vi "Test Decoding Data.vi"() -> ()   [LabVIEW 2019]
uses:
  <vilib>/Analysis/3filter.llb/Filter Passband Type.ctl
  <vilib>/Utility/file.llb/Read Delimited Spreadsheet (DBL).vi
  <vilib>/Analysis/3filter.llb/Elliptic Filter (DBL).vi
  <vilib>/Analysis/NI_AALBase.lvlib
panel:
  out "first row":dbl[](array[numeric])
  out "Rebuild values":dbl[][](array[numeric])
  out "all rows":dbl[][](array[numeric])
  out "Filtered Graph":dbl[](graph)
  in  "ch":i32=1
  out "Original Graph":dbl[](graph)
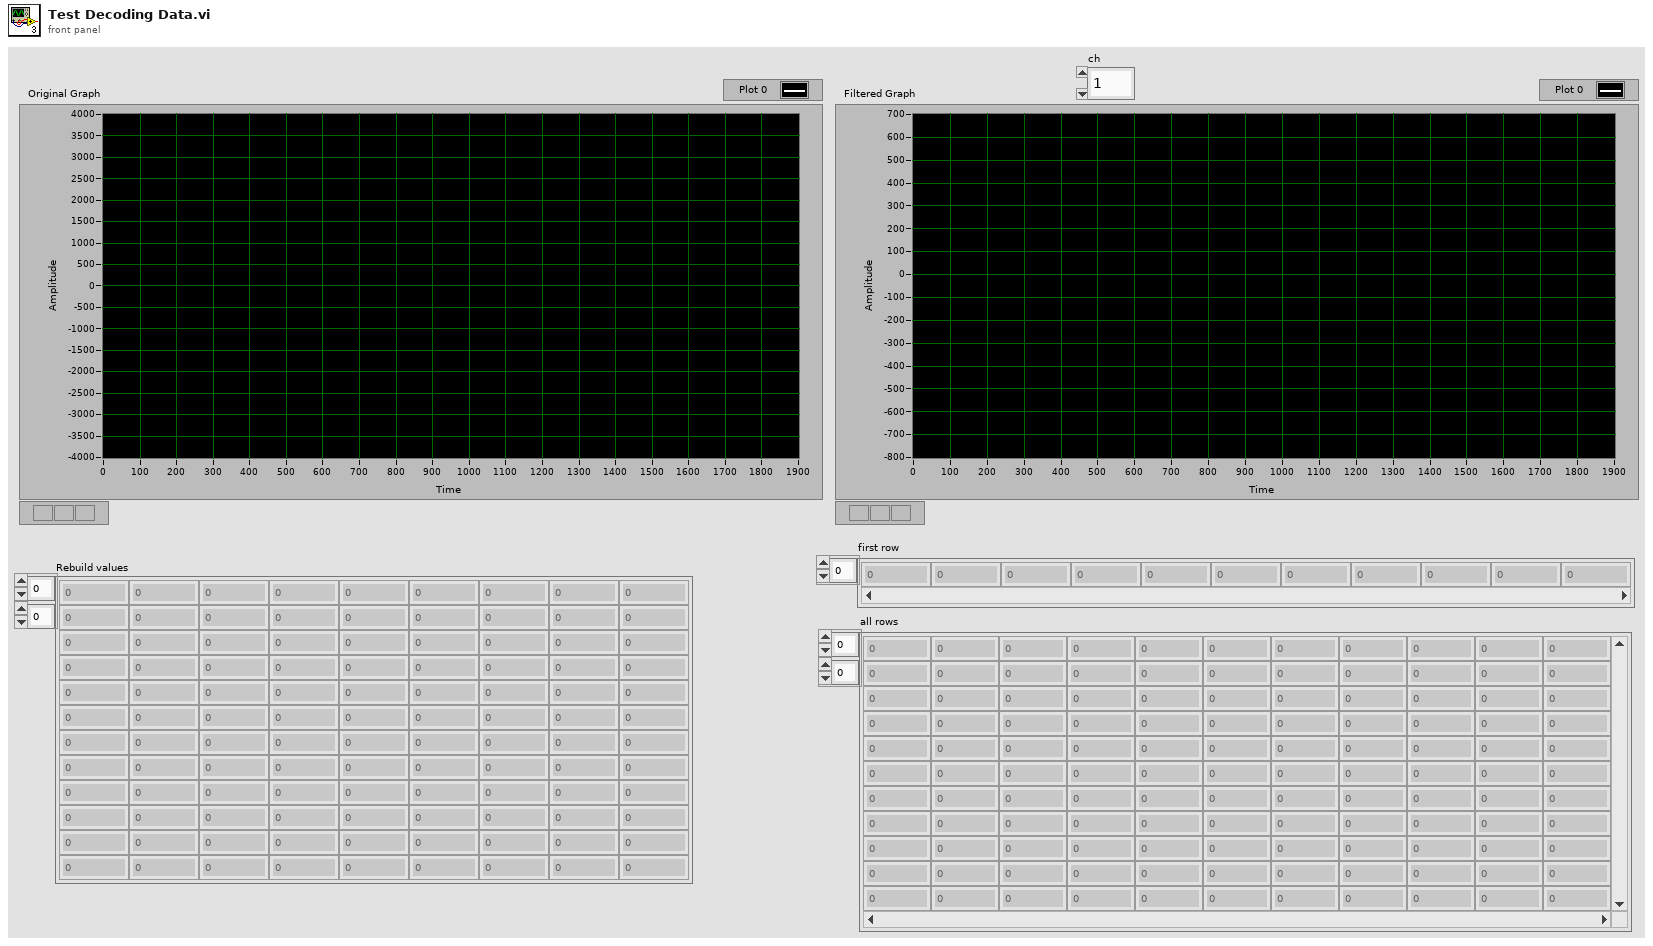
[diagram p1: front panel]
types:
  T1 = typedef "NI_AALBase.lvlib/Filter Passband Type.ctl" = enum32{"Lowpass", "Highpass", "Bandpass", "Bandstop"}
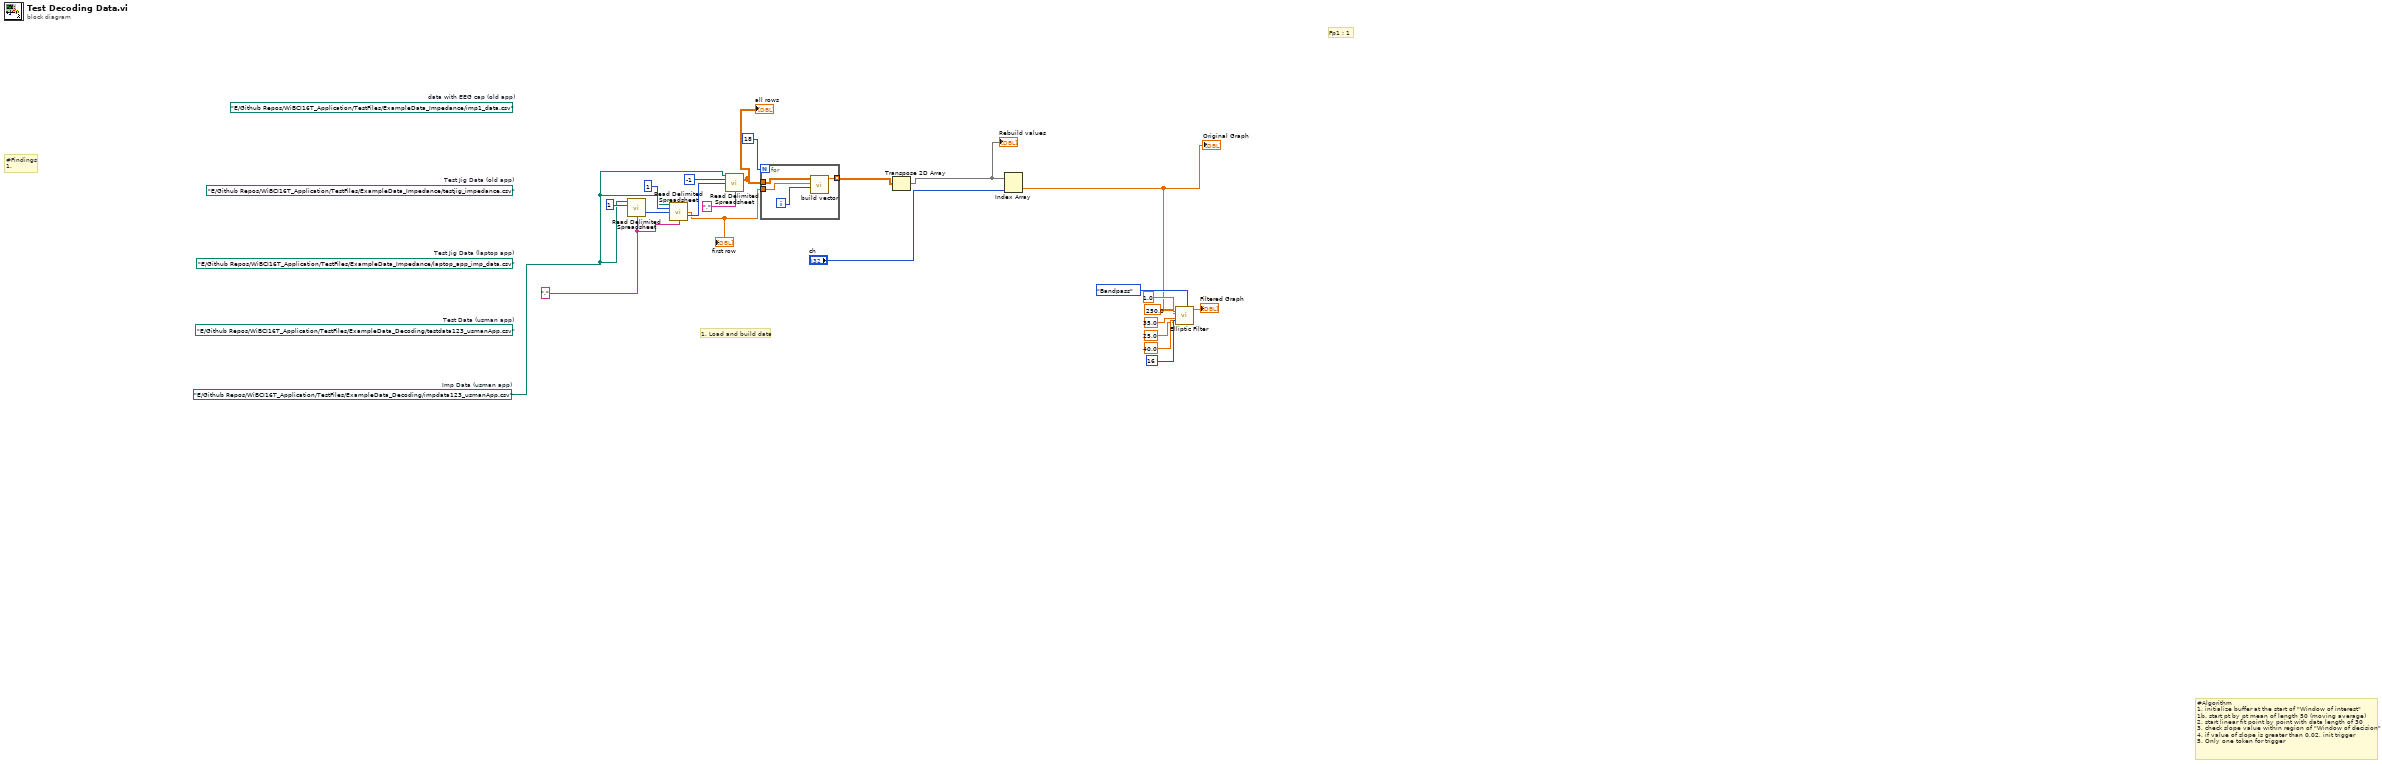
[diagram p0: block diagram]
diagram:
  w1 = path "E:/Github Repos/WiBCI16T_Application/TestFiles/ExampleData_Decoding/impdata123_usmanApp.csv"  # Imp Data (usman app)
  (unwired) path "E:/Github Repos/WiBCI16T_Application/TestFiles/ExampleData_Decoding/testdata123_usmanApp.csv"  # Test Data (usman app)
  (unwired) path "E:/Github Repos/WiBCI16T_Application/TestFiles/ExampleData_Impedance/laptop_app_imp_data.csv"  # Test Jig Data (laptop app)
  (unwired) path "E:/Github Repos/WiBCI16T_Application/TestFiles/ExampleData_Impedance/testjig_impedance.csv"  # Test Jig Data (old app)
  w6 = ","
  (unwired) path "E:/Github Repos/WiBCI16T_Application/TestFiles/ExampleData_Impedance/imp1_data.csv"  # data with EEG cap (old app)
  # "#Findings\n1."
  # "1. Load and build data"
  # "Fp1 : 1"
  # "#Algorithm\n1. initialize buffer at the start of \"Window of interest\"\n1b. start pt by pt mean of length 50 (moving average)\n2. start linear fit point by point with data length of 30\n3. check slope value within region of \"Window of decision\"\n4. if value of slope is greater than 0.02, init trigger\n5. Only one token for trigger"
  n1 = call-poly <vilib>:"Read Delimited Spreadsheet.vi"("file path (dialog if empty)"=w1, "number of rows (all:-1)"=1, "delimiter (\\t)"=w6) -> ("mark after read (chars.)"=w21:i32)  [unwired: 7 in, 5 out]
  n2 = call-poly <vilib>:"Read Delimited Spreadsheet.vi"("file path (dialog if empty)"=w1, "number of rows (all:-1)"=1, "start of read offset (chars.:0)"=w21, "delimiter (\\t)"=w6) -> ("first row"=w5:dbl[], "mark after read (chars.)"=w16:i32)  [unwired: 6 in, 4 out]
  "first row" <- w5
  n3 = call-poly <vilib>:"Read Delimited Spreadsheet.vi"("file path (dialog if empty)"=w1, "number of rows (all:-1)"=-1, "start of read offset (chars.:0)"=w16, "delimiter (\\t)"=",") -> ("all rows"=w18:dbl[][])  [unwired: 6 in, 5 out]
  "all rows" <- w18
  n4 = for {
    N: 18 -> [_]
    tunnel: w18 -> [w27]
    tunnel: w5 -> [w26]
    tunnel: [w25] -> w4 mode=indexing
    i -> [w24]
    n5 = call "build vector.vi"("Index"=w24, "first row"=w26, "diff data"=w27) -> ("Rebuild Vector"=w25:dbl[])  [unwired: 8 in]
  }
  n6 = Transpose 2D Array(2D array=w4) -> (transposed array=w3:dbl[][])
  "Rebuild values" <- w3
  n7 = Index Array(array=w3, index (col)="ch") -> (element=w7:dbl[])  [unwired: 1 in]
  "Original Graph" <- w7
  n8 = call-poly <vilib>:"Elliptic Filter.vi"("order"=16, "filter type"=Filter_Passband_Type."Bandpass", "stopband attenuation (dB)"=40.0, "passband ripple (dB)"=1.0, "low cutoff freq: fl"=25.0, "high cutoff freq: fh"=35.0, "sampling freq: fs"=250.0, "X"=w7) -> ("Filtered X"=→"Filtered Graph":dbl[])  [unwired: 2 in, 1 out]
